vi "OpenVisualizations.vi"(5 "ModuleID":i32, 7 "INIFilePath":path, 8 "ErrorArray in":errorcluster[](array[cluster]), 10 "Module Name (e.g. Sensor.RoomAlert.Model-4E)":string, 11 "Visualization VI Path":path) -> (0 "ErrorArray out":errorcluster[](array[cluster]))   [LabVIEW 2018]
uses:
  VisualizationManagement/VisualizationManagerActions.ctl
  VisualizationManagement/OpenVisualizationVIs.ctl
  <userlib>/NIST/NISTErrorLib/NISTErrorLib.lvlib
  NistPluggableModules/Visualization/VisualizeBase/VisualizeBase_class/VisualizeBase.lvclass
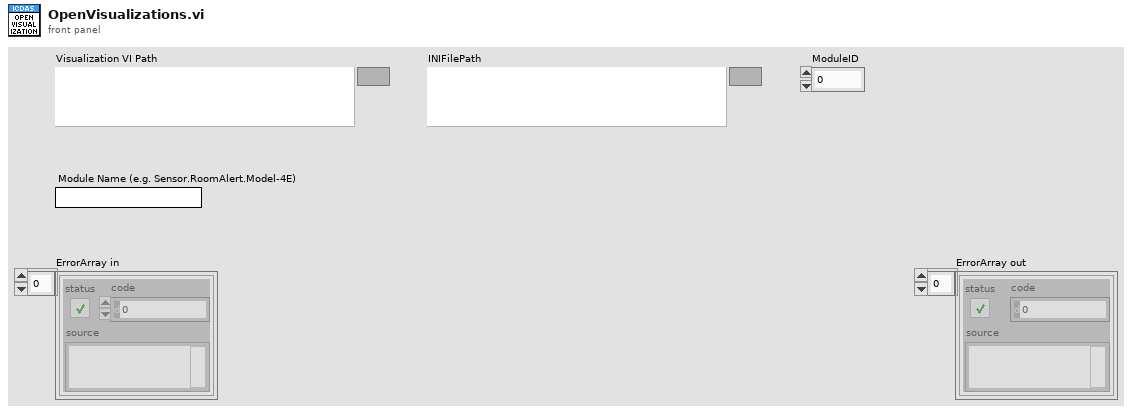
[diagram p1: front panel]
types:
  T1 = typedef "OpenVisualizationVIs.ctl" = cluster{"Module Name":string, "VI ref":refnum<vi>, "In SubPanel?":bool, "Time Stamp":timestamp}
  T2 = typedef "VisualizationManagerActions.ctl" = enum16{"Set", "LoadModVI", "PopInOutModVI", "Add", "Clear", "CloseVisMod", "LoadLatestModule", "Get"}
  T3 = typedef "Visualization.lvlib/VisualizeBase.lvclass/VisualizationOptions.ctl" = cluster{"PauseAtStartup":bool, "LogData":bool, "LaunchInSubPanel":bool, "FPMonitor":u16, "FPWindowBounds":T4, "MonitorBounds":cluster{"Left":i16, "Top":i16, "Right":i16, "Bottom":i16}}
  T4 = typedef "LVRectTypeDef.ctl" = cluster{"Left":i16, "Top":i16, "Right":i16, "Bottom":i16}
  T5 = typedef "cntlRefs.ctl" = cluster{"rngFGen":refnum<vi>, "rngDigitizer":refnum<vi>, "btnHide":refnum<vi>, "rngInst":refnum<vi>, "PluginTree":refnum<vi>, "TestListboxRef":refnum<vi>, "path.tstFile":refnum<vi>, "cmbxRunningModules":refnum<vi>, "TestDataSubPanel":refnum<vi>, "TestDataCaption":refnum<vi>, "btnPopInOut":refnum<vi>, "PluginMgrQ":refnum<queue>, "TestMgrQ":refnum<queue>, "TestMgrSubPanel":refnum<vi>, "PluginMgrSubPanel":refnum<vi>, "PwrReqHandle":u32, "btnStopOneTest":refnum<vi>, "pathUserfiles":refnum<vi>, "PluginTreeCaption":refnum<vi>, "MainVIRef":refnum<vi>, "btnStatus":refnum<vi>}
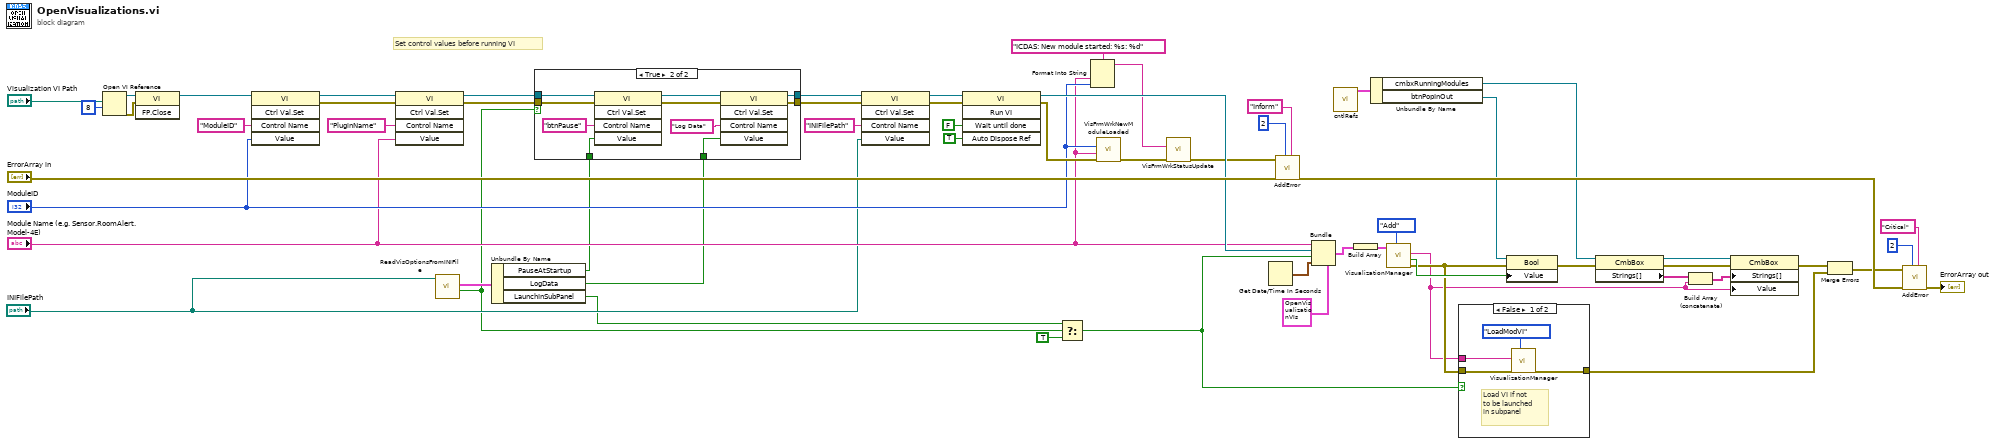
[diagram p0: block diagram]
diagram:
  # "Set control values before running VI"
  n1 = Open VI Reference(vi path="Visualization VI Path", options=8) -> (vi reference=w45:refnum<vi>, error out=w47:errorcluster)  [unwired: 4 in]
  n2 = invoke class="VI" method="FP.Close"(reference=w45, error in=w47) -> (reference out=w29:refnum<vi>)  [unwired: 1 in, 2 out]
  n3 = invoke class="VI" method="Ctrl Val.Set"(reference=w29, "Control Name"="ModuleID", "Value"="ModuleID") -> (reference out=w32:refnum<vi>, error out=w33:errorcluster)  [unwired: 2 in, 3 out]
  n4 = invoke class="VI" method="Ctrl Val.Set"(reference=w32, error in=w33, "Control Name"="PluginName", "Value"="Module Name (e.g. Sensor.RoomAlert.Model-4E)") -> (reference out=w20:refnum<vi>, error out=w19:errorcluster)  [unwired: 1 in, 3 out]
  n5 = call "ReadVisOptionsFromINIFile.vi"("INI File Path"="INIFilePath") -> ("all found?"=w9:bool, "Visualization Properties"=w14:T3)  [unwired: 8 in, 1 out]
  n6 = Unbundle By Name(w14) -> ("PauseAtStartup"=w13:bool, "LogData"=w12:bool, "LaunchInSubPanel"=w8:bool)
  n7 = case shown="True" w9 {
    tunnel: w20 -> [w62 w70]
    tunnel: w19 -> [w61 w69]
    tunnel: [w62 w66] -> w18
    tunnel: [w61 w65] -> w17
    tunnel: w13 -> [_ w64]
    tunnel: w12 -> [_ w63]
    frame False {
    }
    frame True {
      n8 = invoke class="VI" method="Ctrl Val.Set"(reference=w70, error in=w69, "Control Name"="btnPause", "Value"=w64) -> (reference out=w68:refnum<vi>, error out=w67:errorcluster)  [unwired: 1 in, 3 out]
      n9 = invoke class="VI" method="Ctrl Val.Set"(reference=w68, error in=w67, "Control Name"="Log Data", "Value"=w63) -> (reference out=w66:refnum<vi>, error out=w65:errorcluster)  [unwired: 1 in, 3 out]
    }
  }
  n10 = invoke class="VI" method="Ctrl Val.Set"(reference=w18, error in=w17, "Control Name"="INIFilePath", "Value"="INIFilePath") -> (reference out=w16:refnum<vi>, error out=w15:errorcluster)  [unwired: 1 in, 3 out]
  n11 = invoke class="VI" method="Run VI"(reference=w16, error in=w15, "Wait until done"=FALSE ("Wait Until Done"), "Auto Dispose Ref"=TRUE ("Auto Dispose Reference")) -> (reference out=w28:refnum<vi>, error out=w27:errorcluster)  [unwired: 1 in, 3 out]
  n12 = Select(t=w8, s=w9, f=TRUE) -> (s? t:f=w5:bool)
  n13 = Format Into String(format string="ICDAS: New module started: %s: %d", "Module Name (e.g. Sensor.RoomAlert.Model-4E)", "ModuleID") -> (resulting string=w21:string)  [unwired: 2 in, 1 out]
  n14 = call "VisFrmWrkNewModuleLoaded.vi"("error in (no error)"=w27, "Module Name"="Module Name (e.g. Sensor.RoomAlert.Model-4E)", "ModuleID"="ModuleID") -> ("error out"=w26:errorcluster)  [unwired: 8 in]
  n15 = call "VisFrmWrkStatusUpdate.vi"("error in (no error)"=w26, "Status"=w21) -> ("error out"=w25:errorcluster)  [unwired: 9 in]
  n16 = Get Date/Time In Seconds() -> (seconds since 1Jan1904=w30:timestamp)
  n17 = call <userlib>:"AddError.vi"("Severity"="Inform", "Priority"=u8 2, "ErrorArray In"="ErrorArray in", "error in (no error)"=w25) -> ("ErrorArray Out"=w54:errorcluster[])  [unwired: 6 in, 1 out]
  n18 = Bundle(cluster=T1 {"Module Name"="", "VI ref"=refnum, "In SubPanel?"=FALSE, "Time Stamp"=timestamp(0 s since 1904-01-01)} ("Open Visualization VIs"), "Module Name"="Module Name (e.g. Sensor.RoomAlert.Model-4E)", "VI ref"=w28, "In SubPanel?"=w5, "Time Stamp"=w30) -> (w58:T1)
  n19 = call "cntlRefs.vi"() -> ("cntlRefs"=w52:T5)  [unwired: 10 in, 1 out]
  n20 = Build Array(w58) -> (w40:T1[])
  n21 = Unbundle By Name(w52) -> ("cmbxRunningModules"=w37:refnum<vi>, "btnPopInOut"=w49:refnum<vi>)
  n22 = call "VisualizationManager.vi"("Action"=VisualizationManagerActions."Add", "Open Visualization VIs in"=w40) -> ("error out"=w6:errorcluster, "In SubPanel?"=w39:bool, "Module Name out"=w4:string)  [unwired: 6 in, 1 out]
  n23 = case shown="False" w5 {
    tunnel: w6 -> [w76 w77]
    tunnel: w4 -> [w75 _]
    tunnel: [w73 w77] -> w2
    frame False {
      # "Load VI if not \nto be launched \nin subpanel"
      n24 = call "VisualizationManager.vi"("Action"=VisualizationManagerActions."LoadModVI", "error in (no error)"=w76, "Module Name"=w75) -> ("error out"=w73:errorcluster)  [unwired: 5 in, 3 out]
    }
    frame True {
    }
  }
  n25 = property class="Bool"(reference=w49, error in=w6, "Value"=w39) -> (error out=w50:errorcluster)  [unwired: 1 out]
  n26 = property class="CmbBox"(reference=w37, error in=w50) -> (reference out=w36:refnum<vi>, error out=w38:errorcluster, "Strings[]"=w35:string[])
  n27 = Build Array (concatenate)(w35, w4) -> (w34:string[])
  n28 = property class="CmbBox"(reference=w36, error in=w38, "Strings[]"=w34, "Value"=w4) -> (error out=w51:errorcluster)  [unwired: 1 out]
  n29 = Merge Errors(w51, w2) -> (w3:errorcluster)
  n30 = call <userlib>:"AddError.vi"("Severity"="Critical", "Priority"=u8 2, "ErrorArray In"=w54, "error in (no error)"=w3) -> ("ErrorArray Out"=→"ErrorArray out":errorcluster[])  [unwired: 6 in, 1 out]
